vi "Add Channel Group RTM.vi"() -> ()   [LabVIEW 2027, in "Embedded Data Logger System Explorer.lvlib"]
uses:
  Embedded Data Logger System Explorer.lvlib
  <vilib>/NI VeriStand/Custom Device API/Custom Device Item Ref.ctl
  <vilib>/NI VeriStand/Custom Device API/Custom Device API.lvlib
  Scripting/Embedded Data Logger Scripting.lvlib
panel:
  in  "Node Ptr":T1 format="%.0x"
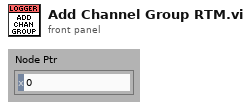
[diagram p1: front panel]
types:
  T1 = typedef "Custom Device API.lvlib/Custom Device Item Ref.ctl" = u64
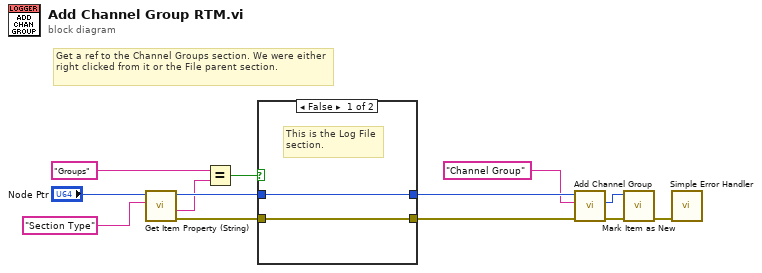
[diagram p0: block diagram]
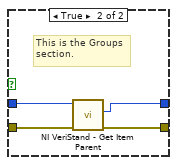
[diagram p2: hidden frame]
diagram:
  # "Get a ref to the Channel Groups section. We were either right clicked from it or the File parent section."
  n1 = call <vilib>:"Get Item Property (String).vi"("Property Name"="Section Type", "Item Ref in"="Node Ptr") -> ("error out"=w6:errorcluster, "Value"=w5:string, "Item Ref out"=w7:T1)  [unwired: 6 in, 1 out]
  n2 = Equal?(x="Groups" ("Property Name"), y=w5) -> (x = y?=w8:bool)
  n3 = case shown="False" w8 {
    tunnel: [w15 w16] -> w13
    tunnel: [w14 w18] -> w12
    tunnel: w7 -> [w15 w17]
    tunnel: w6 -> [w14 w19]
    frame False {
      # "This is the Log File\nsection."
    }
    frame True {
      # "This is the Groups\nsection."
      n4 = call <vilib>:"NI VeriStand - Get Item Parent.vi"("error in (no error)"=w19, "Item Ref in"=w17) -> ("error out"=w18:errorcluster, "Parent Ref"=w16:T1)  [unwired: 6 in, 2 out]
    }
  }
  n5 = call "Add Channel Group.vi"("error in"=w12, "group name"="Channel Group", "log file in"=w13) -> ("error out"=w4:errorcluster, "channel group"=w1:T1)  [unwired: 6 in, 1 out]
  n6 = call "Mark Item as New.vi"("error in (no error)"=w4, "Item Ref in"=w1) -> ("error out"=w2:errorcluster)  [unwired: 8 in, 1 out]
  n7 = call <vilib>:"Simple Error Handler.vi"("error in (no error)"=w2) -> ()  [unwired: 4 in, 5 out]
